vi "Find New Endpoint.vi"(7 "OldVal":i32, 10 "NewVal":i32, 11 "Heights":i32[](array[numeric])) -> (2 "Index":i32, 3 "Endpoint":i32)   [LabVIEW 2018, in "OOPanel.lvlib" / "PanelArray.lvclass"]
uses:
  PanelArray.lvclass
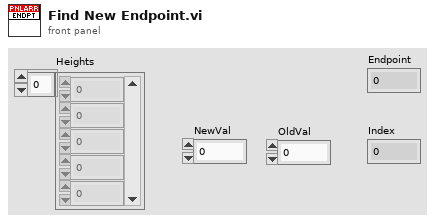
[diagram p1: front panel]
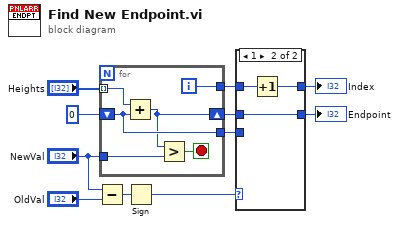
[diagram p0: block diagram]
diagram:
  n1 = Subtract(x="NewVal", y="OldVal") -> (x-y=w4:i32)
  n2 = for {
    tunnel: "Heights" -> [w13] mode=indexing
    tunnel: "NewVal" -> [w17]
    tunnel: [w15] -> w6
    shift-right: [w12] -> w9
    shift-left: 0 -> [w14]
    tunnel: [w14] -> w8
    i -> [w15]
    stop <- w16 stop-if-true
    n3 = Add(x=w13, y=w14) -> (x+y=w12:i32)
    n4 = Greater?(x=w12, y=w17) -> (0:w16:bool)
  }
  n5 = Sign(1:w4) -> (0:w3:i32)
  n6 = case shown="1" w3 {
    tunnel: w9 -> [_ w22]
    tunnel: w8 -> [w18 _]
    tunnel: [w18 w22] -> w7
    tunnel: w6 -> [w19 w21]
    tunnel: [w19 w20] -> w5
    frame Default {
    }
    frame 1 {
      n7 = Increment(x=w21) -> (x+1=w20:i32)
    }
  }
  "Endpoint" <- w7
  "Index" <- w5
